vi "File_ListMenues.vi"(1 "Folder path":path, 5 "error in (no error)":errorcluster) -> (15 "Menues":path[](array[path]), 19 "error out":errorcluster)   [LabVIEW 2020]
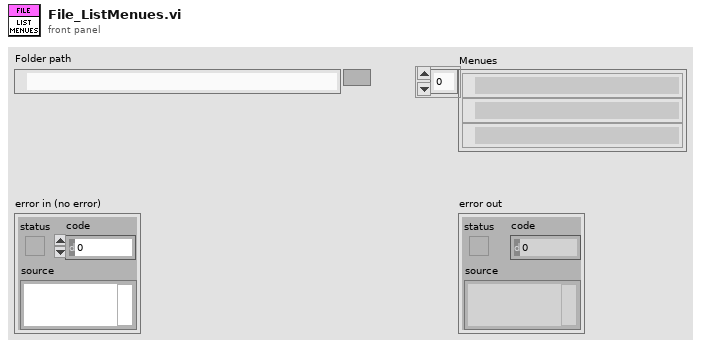
[diagram p1: front panel]
types:
  T1 = typedef "Librarian File List.ctl" = cluster{"name":string, "create date":u32, "mod date":u32, "type":string, "creator":string, "LV version":i32}[]
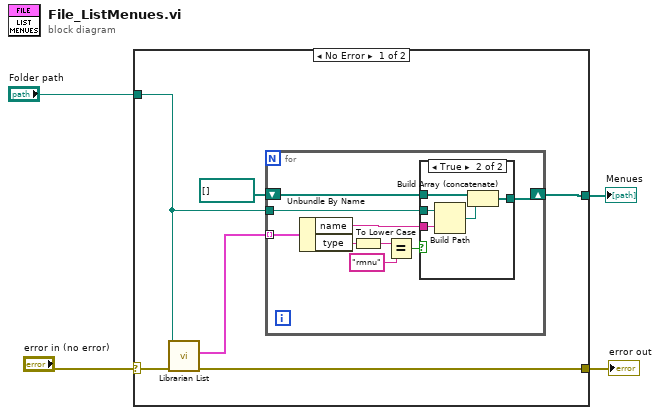
[diagram p0: block diagram]
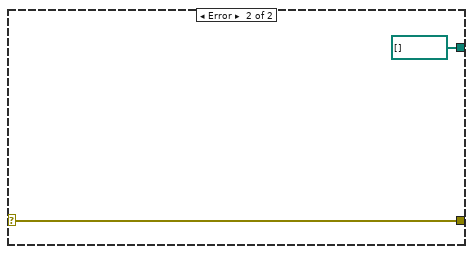
[diagram p3: hidden frame]
diagram:
  n1 = case shown="No Error" "error in (no error)" {
    selector: "error in (no error)" -> [w5 w27]
    tunnel: "Folder path" -> [w8 _]
    tunnel: [w7 w27] -> w3
    tunnel: [w6 path[] [] ("Array Constant")] -> w2
    frame No Error {
      n2 = call <vilib>:"Librarian List.vi"("error in"=w5, "path"=w8) -> ("error out"=w7:errorcluster, "file list"=w10:T1)  [unwired: 8 out]
      n3 = for {
        tunnel: w10 -> [w19] mode=indexing
        shift-right: [w13] -> w6
        shift-left: path[] [] ("Array Constant") -> [w14]
        tunnel: w8 -> [w11]
        n4 = Unbundle By Name(w19) -> ("name"=w12:string, "type"=w18:string)
        n5 = To Lower Case(string=w18) -> (all lower case string=w17:string)
        n6 = Equal?(x=w17, y="rmnu") -> (x = y?=w15:bool)
        n7 = case shown="True" w15 {
          tunnel: w14 -> [w20 w25]
          tunnel: [w20 w24] -> w13
          tunnel: w12 -> [_ w23]
          tunnel: w11 -> [_ w21]
          frame False {
          }
          frame True {
            n8 = Build Path(base path=w21, name or relative path=w23) -> (appended path=w22:path)
            n9 = Build Array (concatenate)(w25, w22) -> (w24:path[])
          }
        }
      }
    }
    frame Error {
    }
  }
  "error out" <- w3
  "Menues" <- w2
